vi "Updated4x7Display.vi"(8 "Error In":errorcluster, 10 "Cluster":cluster{"Score":u32, "Time":u32, "Combo":u32}={"Score"=4, "Time"=4, "Combo"=4}, 11 "LINX Resource In":T1) -> (0 "Error Out":errorcluster, 3 "LINX Resource Out":T1)   [LabVIEW 2022 SP3]
doc: "Custom Command 7 is for the Score Display. Custom Command 8 is for the Time Display. Custom Command 9 is for Combo Display. Sends number to display to the applicable 7 segment display."
uses:
  <vilib>/MakerHub/LINX/Private/Type Defs/LINX Ref.ctl
  <vilib>/MakerHub/LINX/Private/Type Defs/Platform.ctl
  <vilib>/MakerHub/LINX/Private/Type Defs/Interface.ctl
  <vilib>/MakerHub/LINX/Private/Device/Type Defs/LINX Device Config.ctl
  <vilib>/MakerHub/LINX/Private/Device/Type Defs/TCP Config.ctl
  <vilib>/MakerHub/LINX/Private/Device/Type Defs/Channels.ctl
  <vilib>/MakerHub/LINX/LMH-LINX.lvlib
  <vilib>/MakerHub/LINX/Private/Device/Device.lvlib
panel:
  out "Response":u8[](array[numeric])
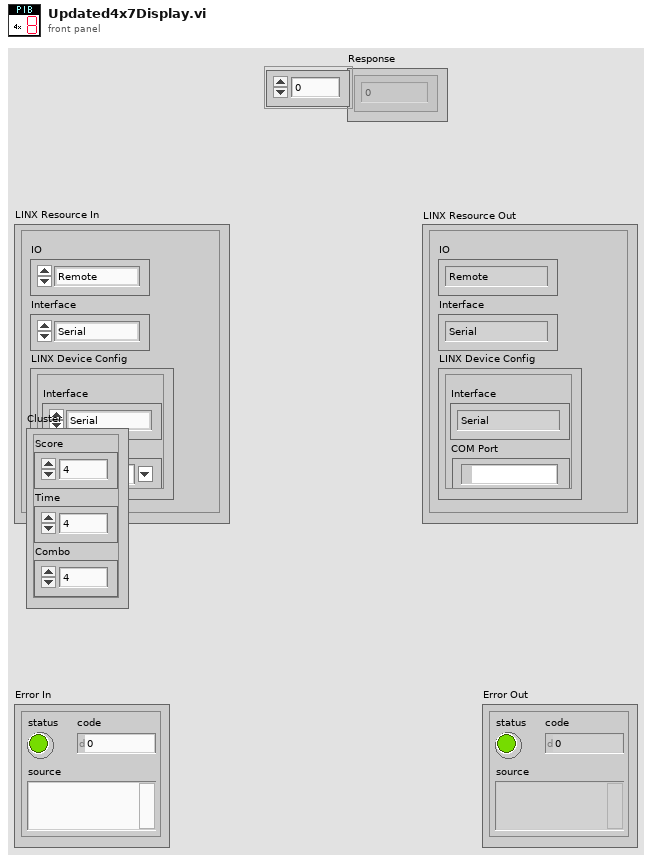
[diagram p1: front panel]
types:
  T1 = typedef "LMH-LINX.lvlib/LINX Ref.ctl" = cluster{"IO":T2, "Interface":T3, "LINX Device Config":T4}
  T2 = typedef "LMH-LINX.lvlib/Platform.ctl" = enum16{"Remote", "Local"}
  T3 = typedef "LMH-LINX.lvlib/Interface.ctl" = enum16{"Serial", "TCP"}
  T4 = typedef "LMH-LINX.lvlib/Device.lvlib/LINX Device Config.ctl" = cluster{"Interface":T3, "COM Port":refnum<visa-resource-name>, "TCP Configuration":T5, "Device Family":u8, "Device ID":u8, "Device Name":string, "TCP Ref":refnum<k5>, "Channels":T6}
  T5 = typedef "LMH-LINX.lvlib/Device.lvlib/TCP Config.ctl" = cluster{"IP Address":string, "Port":u16}
  T6 = typedef "LMH-LINX.lvlib/Channels.ctl" = cluster{"DI":u8[], "DO":u8[], "AI":u8[], "AO":u8[], "PWM":u8[], "QE":u8[], "UART":u8[], "I2C 2":u8[], "SPI":u8[], "CAN":u8[], "Servo":u8[], "AI Ref (V)":dbl, "AI Resolution (Bits)":u8, "AO Ref (V)":dbl, "AO Resolution (Bits)":u8}
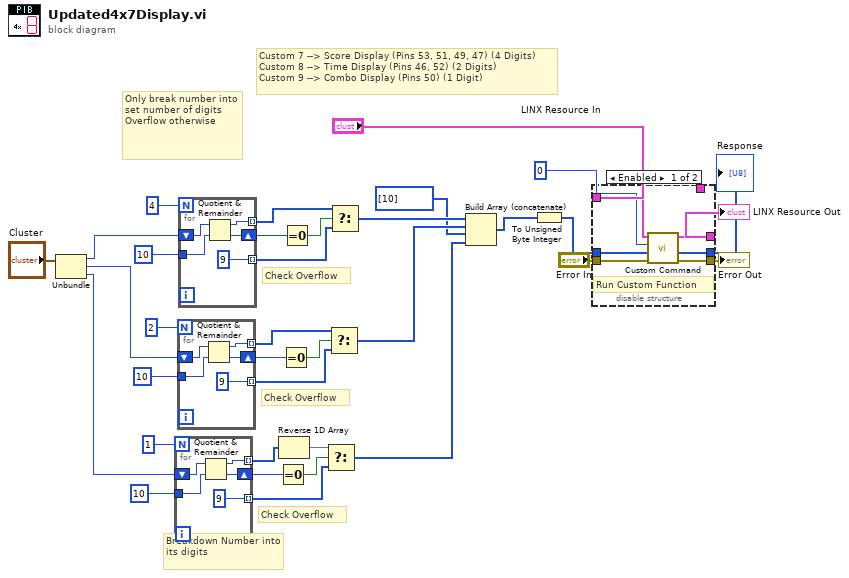
[diagram p0: block diagram]
diagram:
  # "Check Overflow"
  # "Check Overflow"
  # "Check Overflow"
  # "Breakdown Number into its digits"
  # "Custom 7 --> Score Display (Pins 53, 51, 49, 47) (4 Digits)\nCustom 8 --> Time Display (Pins 46, 52) (2 Digits)\nCustom 9 --> Combo Display (Pins 50) (1 Digit)"
  # "Only break number into set number of digits\nOverflow otherwise"
  n1 = Unbundle("Cluster") -> ("Score"=w29:u32, "Time"=w28:u32, "Combo"=w27:u32)
  n2 = for {
    N: 1 ("Display Length") -> [_]
    tunnel: u32 10 -> [w36]
    tunnel: [w38] -> w8 mode=indexing
    tunnel: [u32 9] -> w9 mode=indexing
    shift-right: [w39] -> w7
    shift-left: w27 -> [w40]
    n3 = Quotient & Remainder(x=w40, y=w36) -> (x-y*floor(x/y)=w38:u32, floor(x/y)=w39:u32)
  }
  n4 = for {
    N: 2 ("Display Length") -> [_]
    tunnel: u32 10 -> [w41]
    tunnel: [w43] -> w1 mode=indexing
    tunnel: [u32 9] -> w15 mode=indexing
    shift-right: [w44] -> w14
    shift-left: w28 -> [w45]
    n5 = Quotient & Remainder(x=w45, y=w41) -> (x-y*floor(x/y)=w43:u32, floor(x/y)=w44:u32)
  }
  n6 = for {
    N: 4 ("Display Length") -> [_]
    tunnel: u32 10 -> [w46]
    tunnel: [w48] -> w2 mode=indexing
    tunnel: [u32 9] -> w20 mode=indexing
    shift-right: [w49] -> w19
    shift-left: w29 -> [w50]
    n7 = Quotient & Remainder(x=w50, y=w46) -> (x-y*floor(x/y)=w48:u32, floor(x/y)=w49:u32)
  }
  n8 = Equal To 0?(x=w7) -> (x = 0?=w10:bool)
  n9 = Reverse 1D Array(array=w8) -> (reversed array=w11:u32[])
  n10 = Equal To 0?(x=w14) -> (x = 0?=w16:bool)
  n11 = Equal To 0?(x=w19) -> (x = 0?=w21:bool)
  n12 = Select(t=w11, s=w10, f=w9) -> (s? t:f=w4:u32[])
  n13 = Select(t=w1, s=w16, f=w15) -> (s? t:f=w22:u32[])
  n14 = Select(t=w2, s=w21, f=w20) -> (s? t:f=w23:u32[])
  n15 = Build Array (concatenate)(w23, w22, u32[] [10] ("array"), w4) -> (w26:u32[])
  n16 = To Unsigned Byte Integer(number=w26) -> (unsigned 8bit integer=w34:u8[])
  n17 = disable-structure shown="Enabled" {
    disable-tunnel: u16 0 ("Custom Command Number") -> [w57 _]
    disable-tunnel: w34 -> [w56 w59]
    disable-tunnel: "LINX Resource In" -> [w55 _]
    disable-tunnel: [w54 w60] -> w33
    disable-tunnel: "Error In" -> [w53 w58]
    disable-tunnel: [w52 w58] -> w31
    disable-tunnel: [w51 w59] -> w25
    disable-tunnel: "LINX Resource In" -> [_ w60]
    frame Enabled {
      # "Run Custom Function"
      n18 = call <vilib>:"Custom Command.vi"("Error In"=w53, "Data"=w56, "Custom Command Number"=w57, "LINX Resource"=w55) -> ("Error Out"=w52:errorcluster, "Response"=w51:u8[], "LINX Resource"=w54:T1)  [unwired: 4 in, 1 out]
    }
    frame Disabled {
    }
  }
  "LINX Resource Out" <- w33
  "Error Out" <- w31
  "Response" <- w25
